vi "PH_AWG-510.Save Settings.vi"(0 "VI in":refnum<vi>, 5 "error in (no error)":errorcluster) -> (14 "VI out":refnum<vi>, 19 "error out":errorcluster)   [LabVIEW 2014, in "PH_AWG-510.lvlib"]
doc: "This VI saves the current settings at harddisk for further use."
uses:
  PH_AWG-510.lvlib
  PH_Common/Names/PH_Names.File Types.ctl
  PH_Common/PH_Common.lvlib
panel:
  in  "Current Settings.Trigger.Mode":T1(ring)
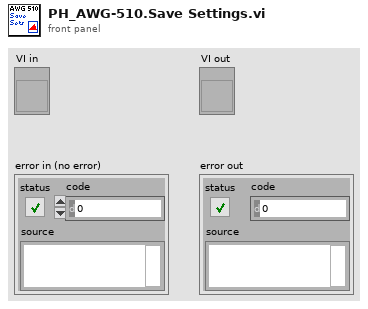
[diagram p1: front panel]
types:
  T1 = enum16{"Continuous", "Triggered", "Gated", "Enhanced"}
  T2 = typedef "PH_Common.lvlib/PH_Names.File Types.ctl" = string
  T3 = typedef "PH_AWG-510.lvlib/PH_AWG-510.i attribute.ctl" = cluster{"GUI Refs":cluster{"Delete":refnum<vi>, "Trigger Settings":refnum<vi>, "Start Device":refnum<vi>, "Instrument Information":refnum<vi>, "Lock Frontpanel":refnum<vi>, "Waveform Pattern File":refnum<vi>, "Initialize":refnum<vi>, "Output Settings":refnum<vi>}, "Instrument Information":T4, "Initialized?":bool, "Current Settings":cluster{"Trigger":T5, "Output Settings":T6}, "Wanted Settings":cluster{"Trigger":T5, "Output Settings":T6}, "Device frontpanel locked?":bool, "Default File Path":path}
  T4 = typedef "PH_AWG-510.lvlib/PH_AWG-510.Instrument Information Dataset.ctl" = cluster{"VISA resource name":refnum<visa-resource-name>, "Instrument Firmware Revision":string, "Manufacturer":string, "Model":string, "Serial Number":string, "Error Message":string, "Device Status":enum16{"stopped", "wating for trigger", "running", "Failure"}}
  T5 = typedef "PH_AWG-510.lvlib/PH_AWG-510.Trigger Settings.ctl" = cluster{"Mode":enum16{"Continuous", "Triggered", "Gated", "Enhanced"}, "Level (V)":dbl, "External Source":bool}
  T6 = typedef "PH_AWG-510.lvlib/PH_AWG-510.Output Settings.ctl" = cluster{"Activate Channel":bool, "VPP (V)":dbl, "Clock (Hz)":dbl, "File Name (Device)":string, "#1":u16, "#2":u16, "#3":u16, "#4":u16, "#5":u16, "#6":u16, "#7":u16, "#8":u16, "#9":u16, "#10":u16, "#11":u16, "#12":u16, "#13":u16, "#14":u16, "#15":u16, "#16":u16, "#17":u16, "#18":u16, "#19":u16, "#20":u16, "Offset (V)":dbl}
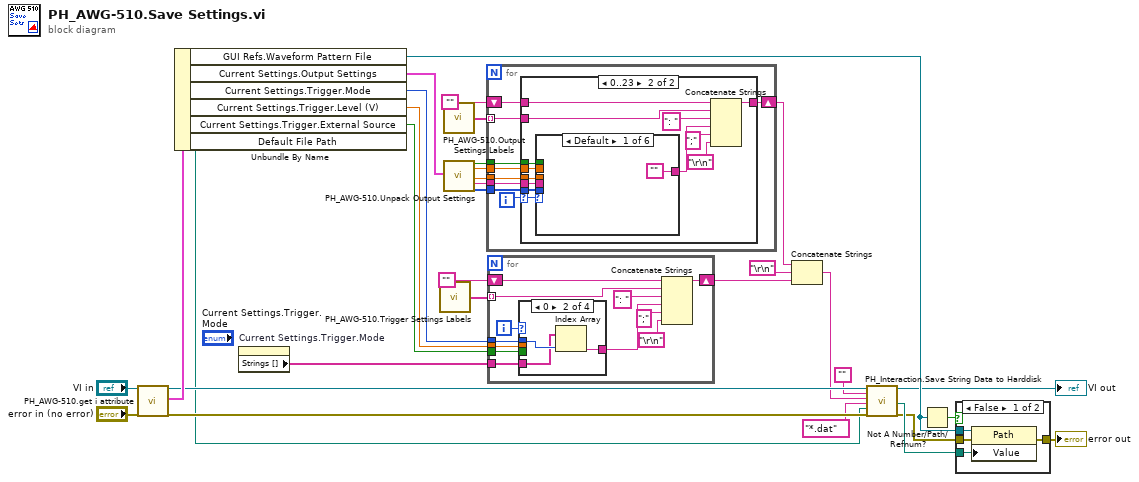
[diagram p0: block diagram]
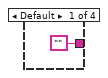
[diagram p2: hidden frame]
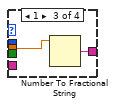
[diagram p3: hidden frame]
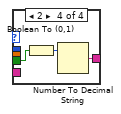
[diagram p4: hidden frame]
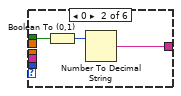
[diagram p6: hidden frame]
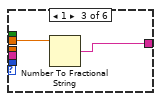
[diagram p7: hidden frame]
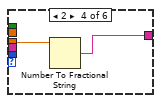
[diagram p8: hidden frame]
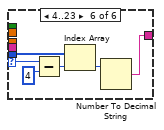
[diagram p10: hidden frame]
diagram:
  n1 = call "PH_AWG-510.get i attribute.vi"("i ref in"="VI in", "error in (no error)"="error in (no error)") -> ("i ref out"=w22:refnum<vi>, "i attribute"=w29:T3, "error out"=w25:errorcluster)  [unwired: 15 in]
  n2 = Unbundle By Name(w29) -> ("GUI Refs.Waveform Pattern File"=w27:refnum<vi>, "Current Settings.Output Settings"=w20:T6, "Current Settings.Trigger.Mode"=w11:T1, "Current Settings.Trigger.Level (V)"=w10:dbl, "Current Settings.Trigger.External Source"=w9:bool, "Default File Path"=w1:path)
  n3 = property on="Current Settings.Trigger.Mode" class="Enum (strict)"() -> ("Strings []"=w2:string[])  [unwired: 2 in, 2 out]
  n4 = call "PH_AWG-510.Trigger Settings Labels.vi"() -> ("Trigger Settings Labels"=w8:string[])
  n5 = call "PH_AWG-510.Output Settings Labels.vi"() -> ("Output Settings Labels"=w19:string[])
  n6 = call "PH_AWG-510.Unpack Output Settings.vi"("Output Settings"=w20) -> ("Activate Channel"=w18:bool, "VPP [V]"=w17:dbl, "Clock [Hz]"=w16:dbl, "File Name (Device)"=w15:string, "Waveform Pattern"=w14:u16[])  [unwired: 14 in]
  n7 = for {
    tunnel: w19 -> [w36] mode=indexing
    tunnel: w18 -> [w40]
    tunnel: w17 -> [w39]
    tunnel: w16 -> [w38]
    tunnel: w15 -> [w37]
    tunnel: w14 -> [w41]
    shift-right: [w35] -> w4
    shift-left: "" -> [w34]
    i -> [w33]
    n8 = case shown="0..23" w33 {
      selector: w33 -> [_ w43]
      tunnel: w41 -> [_ w55]
      tunnel: w40 -> [_ w53]
      tunnel: w39 -> [_ w52]
      tunnel: w38 -> [_ w51]
      tunnel: w37 -> [_ w50]
      tunnel: w36 -> [_ w49]
      tunnel: [w42 w45] -> w35
      tunnel: w34 -> [w42 w44]
      frame Default {
      }
      frame 0..23 {
        n9 = case shown="Default" w43 {
          selector: w43 -> [_ _ _ _ _ w67]
          tunnel: w55 -> [_ _ _ _ _ w70]
          tunnel: w53 -> [_ w59 _ _ _ _]
          tunnel: w52 -> [_ _ w60 _ _ _]
          tunnel: w51 -> [_ _ _ w62 _ _]
          tunnel: w50 -> [_ _ _ _ w64 _]
          tunnel: ["" w57 w61 w63 w64 w69] -> w48
          frame Default {
          }
          frame 0 {
            n10 = Boolean To (0,1)(Boolean=w59) -> (0, 1=w58:i16)
            n11 = Number To Decimal String(number=w58) -> (decimal integer string=w57:string)  [unwired: 1 in]
          }
          frame 1 {
            n12 = Number To Fractional String(number=w60) -> (F-format string=w61:string)  [unwired: 3 in]
          }
          frame 2 {
            n13 = Number To Fractional String(number=w62) -> (F-format string=w63:string)  [unwired: 3 in]
          }
          frame 3 {
          }
          frame 4..23 {
            n14 = Subtract(x=w67, y=4) -> (x-y=w66:i32)
            n15 = Index Array(array=w70, index=w66) -> (element=w68:u16)
            n16 = Number To Decimal String(number=w68) -> (decimal integer string=w69:string)  [unwired: 1 in]
          }
        }
        n17 = Concatenate Strings(w44, w49, ": " ("string"), w48, ";" ("string"), "\r\n") -> (w45:string)
      }
    }
  }
  n18 = for {
    tunnel: w8 -> [w77] mode=indexing
    tunnel: w11 -> [w80]
    tunnel: w10 -> [w79]
    tunnel: w9 -> [w78]
    shift-right: [w73] -> w5
    shift-left: "" -> [w72]
    tunnel: w2 -> [w71]
    i -> [w82]
    n19 = case shown="0" w82 {
      tunnel: w80 -> [_ w85 _ _]
      tunnel: w79 -> [_ _ w87 _]
      tunnel: w78 -> [_ _ _ w89]
      tunnel: ["" w86 w88 w90] -> w76
      tunnel: w71 -> [_ w84 _ _]
      frame Default {
      }
      frame 0 {
        n20 = Index Array(array=w84, index=w85) -> (element=w86:string)
      }
      frame 1 {
        n21 = Number To Fractional String(number=w87) -> (F-format string=w88:string)  [unwired: 3 in]
      }
      frame 2 {
        n22 = Boolean To (0,1)(Boolean=w89) -> (0, 1=w91:i16)
        n23 = Number To Decimal String(number=w91) -> (decimal integer string=w90:string)  [unwired: 1 in]
      }
    }
    n24 = Concatenate Strings(w72, w77, ": " ("string"), w76, ";" ("string"), "\r\n") -> (w73:string)
  }
  n25 = Concatenate Strings(w4, "\r\n", w5) -> (w3:string)
  n26 = call "PH_Interaction.Save String Data to Harddisk.vi"("i ref in"=w22, "Explanation (for Example: Column 1: xxx, ...)"="", "Data (for example: Columns)"=w3, "file name extension"=T2 "*.dat", "start path (O:\\)"=w1, "error in (no error)"=w25) -> ("i ref out"=→"VI out":refnum<vi>, "File Path"=w26:path, "error out"=w24:errorcluster)  [unwired: 11 in]
  n27 = Not A Number/Path/Refnum?(number/path/refnum=w27) -> (NaN/Path/Refnum?=w28:bool)
  n28 = case shown="False" w28 {
    tunnel: w24 -> [w95 w96]
    tunnel: [w94 w96] -> w30
    tunnel: w27 -> [w93 _]
    tunnel: w26 -> [w92 _]
    frame False {
      n29 = property class="Path"(reference=w93, error in=w95, "Value"=w92) -> (error out=w94:errorcluster)  [unwired: 1 out]
    }
    frame True {
    }
  }
  "error out" <- w30
